vi "SetAttributeViReal64_SS-DMod_ListSeq_RF.vi"(0 "instrument handle":refnum<k15>, 1 "AttributeValue":dbl, 2 "AttributeID":u32(ring)=1150887 items=["SS_DIGITALMODULATION_ARB_EXTERNAL_TRIGGER_DELAY"=1150887, "SS_DIGITALMODULATION_ARB_IQADJUSTMENT_DELAY"=1150920, "SS_DIGITALMODULATION_ARB_IQADJUSTMENT_GAIN"=1150919, "SS_DIGITALMODULATION_ARB_RMS_VALUE"=1150891, "SS_DIGITALMODULATION_ARB_RUN_TIME_SCALING"=1150880, "SS_DIGITALMODULATION_ARB_SAMPLING_RATE"=1150890, "SS_DIGITALMODULATION_BASE_FREQUENCY_OFFSET"=1150889, "SS_RFGENERATOR_FREQUENCY"=1150922, "SS_RFGENERATOR_LEVEL"=1150924, "SS_RFGENERATOR_MODULATION_AM_DEPTH"=1150926, "SS_RFGENERATOR_MODULATION_AM_FREQUENCY"=1150928, "SS_RFGENERATOR_MODULATION_ANALOG_DUTY_CYCLE"=1150937, "SS_RFGENERATOR_MODULATION_ANALOG_SINE2_FREQUENCY"=1150939, "SS_RFGENERATOR_MODULATION_ANALOG_SINE2_LEVEL"=1150938, "SS_RFGENERATOR_MODULATION_FM_DEVIATION"=1150929, "SS_RFGENERATOR_MODULATION_FM_FREQUENCY"=1150931, "SS_RFGENERATOR_MODULATION_PM_DEVIATION"=1150934, "SS_RFGENERATOR_MODULATION_PM_FREQUENCY"=1150933, "SS_RFGENERATOR_OFFSET_FREQUENCY"=1150923, "SS_RFGENERATOR_OFFSET_POWER"=1150916, "SS_RFGENERATOR_REFERENCE_FREQUENCY"=1150912, "SS_RFGENERATOR_REFERENCE_POWER"=1150914], 3 "error in (no error)":errorcluster {"code" format="%.0x"}) -> (7 "instrument handle out":refnum<k15>, 10 "error out":errorcluster {"code" format="%.0x"})   [LabVIEW 2009, in "Keysight XSAn.lvlib"]
doc: "Sets a Real64 attribute from the instrument driver.\nThe following Attributes are supported:\n\nSS_DIGITALMODULATION_ARB_EXTERNAL_TRIGGER_DELAY\nSS_DIGITALMODULATION_ARB_IQADJUSTMENT_DELAY\nSS_DIGITALMODULATION_ARB_IQADJUSTMENT_GAIN\nSS_DIGITALMODULATION_ARB_RMS_VALUE\nSS_DIGITALMODULATION_ARB_RUN_TIME_SCALING\nSS_DIGITALMODULATION_ARB_SAMPLING_RATE\nSS_DIGITALMODULATION_BASE_FREQUENCY_OFFSET\nSS_RFGENERATOR_FREQUENCY\nSS_RFGENERATOR_LEVEL\nSS_RFGENERATOR_MODULATION_AM_DEPTH\nSS_RFGENERATOR_MODULATION_AM_FREQUENCY\nSS_RFGENERATOR_MODULATION_ANALOG_DUTY_CYCLE\nSS_RFGENERATOR_MODULATION_ANALOG_SINE2_FREQUENCY\nSS_RFGENERATOR_MODULATION_ANALOG_SINE2_LEVEL\nSS_RFGENERATOR_MODULATION_FM_DEVIATION\nSS_RFGENERATOR_MODULATION_FM_FREQUENCY\nSS_RFGENERATOR_MODULATION_PM_DEVIATION\nSS_RFGENERATOR_MODULATION_PM_FREQUENCY\nSS_RFGENERATOR_OFFSET_FREQUENCY\nSS_RFGENERATOR_OFFSET_POWER\nSS_RFGENERATOR_REFERENCE_FREQUENCY\nSS_RFGENERATOR_REFERENCE_POWER"
uses:
  <instrlib>/Keysight XSAn/Keysight XSAn.lvlib
  AgXSAn.dll
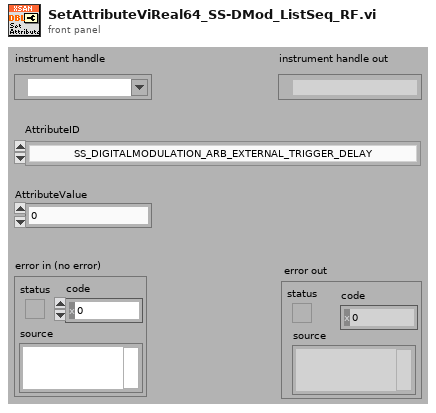
[diagram p1: front panel]
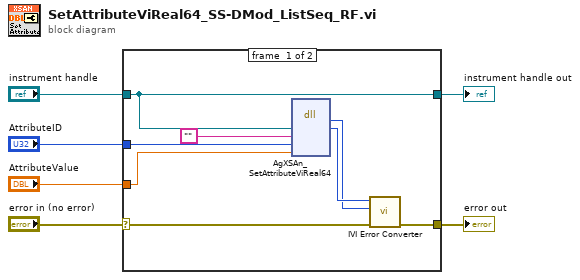
[diagram p0: block diagram]
diagram:
  n1 = case shown="No Error" "error in (no error)" {
    selector: "error in (no error)" -> [w12 w16]
    tunnel: [w11 w16] -> w6
    tunnel: "instrument handle" -> [w8 w15]
    tunnel: "AttributeID" -> [w10 _]
    tunnel: "AttributeValue" -> [w9 _]
    tunnel: [w8 w15] -> w2
    frame #0 {
      n2 = dll-call lib="AgXSAn**.dll" fn="AgXSAn_SetAttributeViReal64"("Vi"=w8, "RepCapIdentifier"="", "AttributeID"=w10, "AttributeValue"=w9) -> ("return type"=w13:i32, "Vi"=w14:u32)  [unwired: 6 in, 2 out]
      n3 = call <instrlib>:"IVI Error Converter.vi"("error in (no error)"=w12, "IVI error code (0)"=w13, "instrument handle"=w14) -> ("error out"=w11:errorcluster)  [unwired: 7 in, 1 out]
    }
    frame #1 {
    }
  }
  "error out" <- w6
  "instrument handle out" <- w2
